vi "Find Msgs.vi"(10 "Actor":refnum<class "Actor.lvclass">) -> (2 "Msgs":T1)   [LabVIEW 2020, in "jettl.lvlib" / "Actor.lvlib"]
uses:
  Actor.lvlib
  Msgs.ctl
  Msg/Msg.lvclass
  Actor/Actor.lvclass
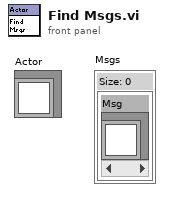
[diagram p1: front panel]
types:
  T1 = typedef "jettl.lvlib/Actor.lvlib/Msgs.ctl" = set{refnum<class "Msg.lvclass">}
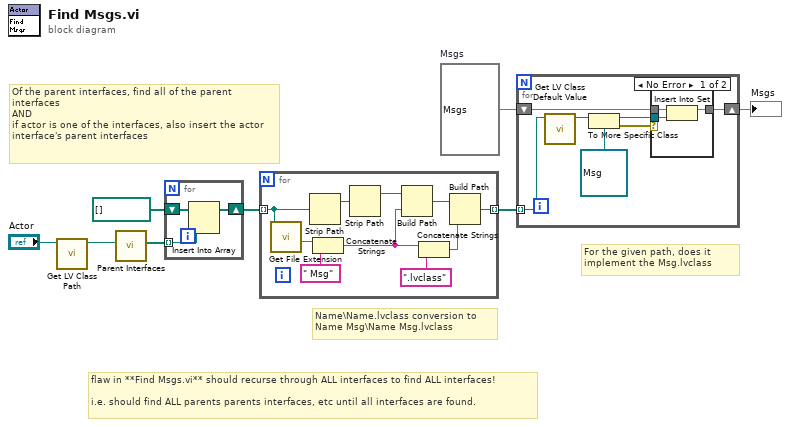
[diagram p0: block diagram]
diagram:
  w5 = T1 {}  # Msgs
  # "flaw in **Find Msgs.vi** should recurse through ALL interfaces to find ALL interfaces!\n\ni.e. should find ALL parents parents interfaces, etc until all interfaces are found."
  # "For the given path, does it implement the Msg.lvclass"
  # "Name\\Name.lvclass conversion to\nName Msg\\Name Msg.lvclass"
  # "Of the parent interfaces, find all of the parent interfaces\nAND\nif actor is one of the interfaces, also insert the actor interface's parent interfaces"
  n1 = call <vilib>:"Get LV Class Path.vi"("object"="Actor") -> ("class path"=w2:path)  [unwired: 9 in, 1 out]
  n2 = call "Parent Interfaces.vi"("Path"=w2) -> ("Parent Interface Paths"=w8:path[])  [unwired: 9 in, 1 out]
  n3 = for {
    tunnel: w8 -> [w9] mode=indexing
    shift-right: [w11] -> w6
    shift-left: path[] [] ("Array 2") -> [w10]
    n4 = Insert Into Array(array=w10, new element=w9) -> (w11:path[])  [unwired: 1 in]
  }
  n5 = for {
    tunnel: w6 -> [w21] mode=indexing
    tunnel: [w17] -> w4 mode=indexing
    n6 = call <vilib>:"Get File Extension.vi"("file"=w21) -> ("filename without extension"=w13:string)  [unwired: 6 in, 4 out]
    n7 = Strip Path(path=w21) -> (stripped path=w20:path)  [unwired: 1 out]
    n8 = Concatenate Strings(w13, " Msg" ("string")) -> (w12:string)
    n9 = Strip Path(path=w20) -> (stripped path=w15:path)  [unwired: 1 out]
    n10 = Build Path(base path=w15, name or relative path=w12) -> (appended path=w14:path)
    n11 = Concatenate Strings(w12, ".lvclass" ("string")) -> (w19:string)
    n12 = Build Path(base path=w14, name or relative path=w19) -> (appended path=w17:path)
  }
  n13 = for {
    shift-right: [w27] -> w3
    shift-left: w5 -> [w28]
    tunnel: w4 -> [w24] mode=indexing
    n14 = call <vilib>:"Get LV Class Default Value.vi"("class path"=w24) -> ("object"=w25:refnum<class>)  [unwired: 9 in, 1 out]
    n15 = To More Specific Class(target class=refnum<class "Msg.lvclass"> refnum ("Msg"), reference=w25) -> (specific class reference=w26:refnum<class "Msg.lvclass">, error out=w22:errorcluster)  [unwired: 1 in]
    n16 = case shown="No Error" w22 {
      tunnel: w28 -> [w31 w32]
      tunnel: [w30 w32] -> w27
      tunnel: w26 -> [w29 _]
      frame No Error {
        n17 = Insert Into Set(10:w29, 11:w31) -> (3:w30:T1)  [unwired: 1 out]
      }
      frame Error {
      }
    }
  }
  "Msgs" <- w3
